vi "Close Connection.vi"(8 "error in (no error)":errorcluster, 11 "RemoteControl.ZMQ in":refnum<class "RemoteControl.ZMQ.lvclass">) -> (0 "error out":errorcluster, 3 "RemoteControl.ZMQ out":refnum<class "RemoteControl.ZMQ.lvclass">)   [LabVIEW 2016, in "RemoteControl.ZMQ.lvclass"]
uses:
  RemoteControl.ZMQ.lvclass
  <vilib>/addons/zeromq/zmq_socket.lvclass
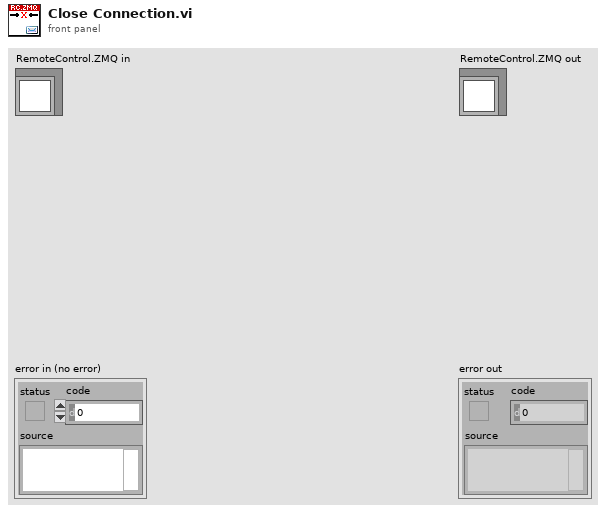
[diagram p1: front panel]
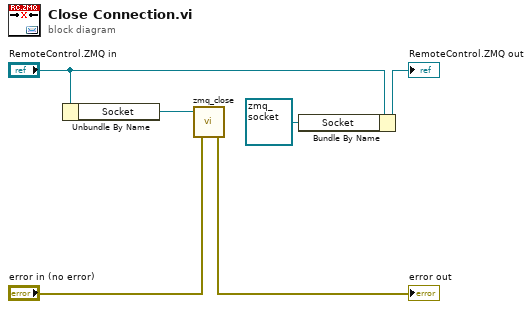
[diagram p0: block diagram]
diagram:
  n1 = Unbundle By Name("RemoteControl.ZMQ in") -> ("Socket"=w6:refnum<class "zmq_socket.lvclass">)
  n2 = call <vilib>:"zmq_close.vi"("error in"="error in (no error)", "socket"=w6) -> ("error out"=→"error out":errorcluster)  [unwired: 3 in]
  n3 = Bundle By Name(cluster="RemoteControl.ZMQ in", "Socket"=refnum<class "zmq_socket.lvclass"> refnum ("socket")) -> (→"RemoteControl.ZMQ out":refnum<class "RemoteControl.ZMQ.lvclass">)
